vi "Color_Data_Logging.vi"   [LabVIEW 2012]
uses:
  <vilib>/NXT/Block Support/NXT_InputPort.ctl
  <vilib>/NXT/Dual Mode Library/Logging/LogRedData_light.vi
  <vilib>/NXT/Dual Mode Library/Display/drawNumber.vi
types:
  T1 = typedef "NXT_InputPort.ctl" = u32
  T2 = typedef "ColorSensorColors.ctl" = enum16{"No Color", "Black", "Blue", "Green", "Yellow", "Red", "White", "Brown"}
  T3 = typedef "LVHSConnector.ctl" = refnum<class "BrickReference.lvclass">
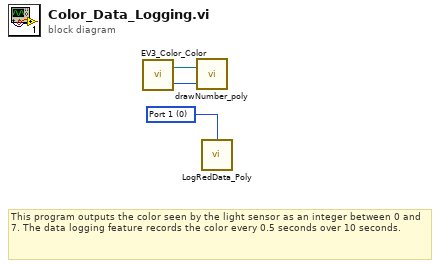
[diagram p0: block diagram]
diagram:
  w1 = T1 0 items=["Port 1", "Port 2", "Port 3", "Port 4"] ("Port (Port 3)")
  # "This program outputs the color seen by the light sensor as an integer between 0 and 7. The data logging feature records the color every 0.5 seconds over 10 seconds."
  n1 = call <vilib>:"EV3_Color_Color.vi"() -> ("Detected Color"=w2:T2, "NXT/EV3"=w3:T3)  [unwired: 3 in]
  n2 = call-poly <vilib>:"drawNumber_poly.vi"("number"=w2, "NXT/EV3"=w3) -> ()  [unwired: 2 in, 1 out]
  n3 = call-poly <vilib>:"LogRedData_Poly.vi"("Port (Port 3)"=w1) -> ()  [unwired: 3 in, 1 out]
